vi "dl.vi"() -> ()   [LabVIEW 2025]
uses:
  <vilib>/Instr/_visa.llb/VISA Configure Serial Port (Instr).vi
panel:
  out "KONDENSATOR":dbl(slide) scale=2.8..3.3
  in  "?":bool
  in  "ILOŒÆ D¯ULI":dbl
  out "OSTATNI LOG":string
  out "LOGI":string[](array[string])
  in  "KONTRAST":dbl(knob) scale=0.0..1000.0
  in  "?":bool
  in  "?":bool
  in  "?":bool
  out "KONDENSATOR":dbl(graph)
  in  "stop":bool
  out "AKTUALNA WARTOŒÆ":dbl
  out "REZYSTOR":dbl(graph)
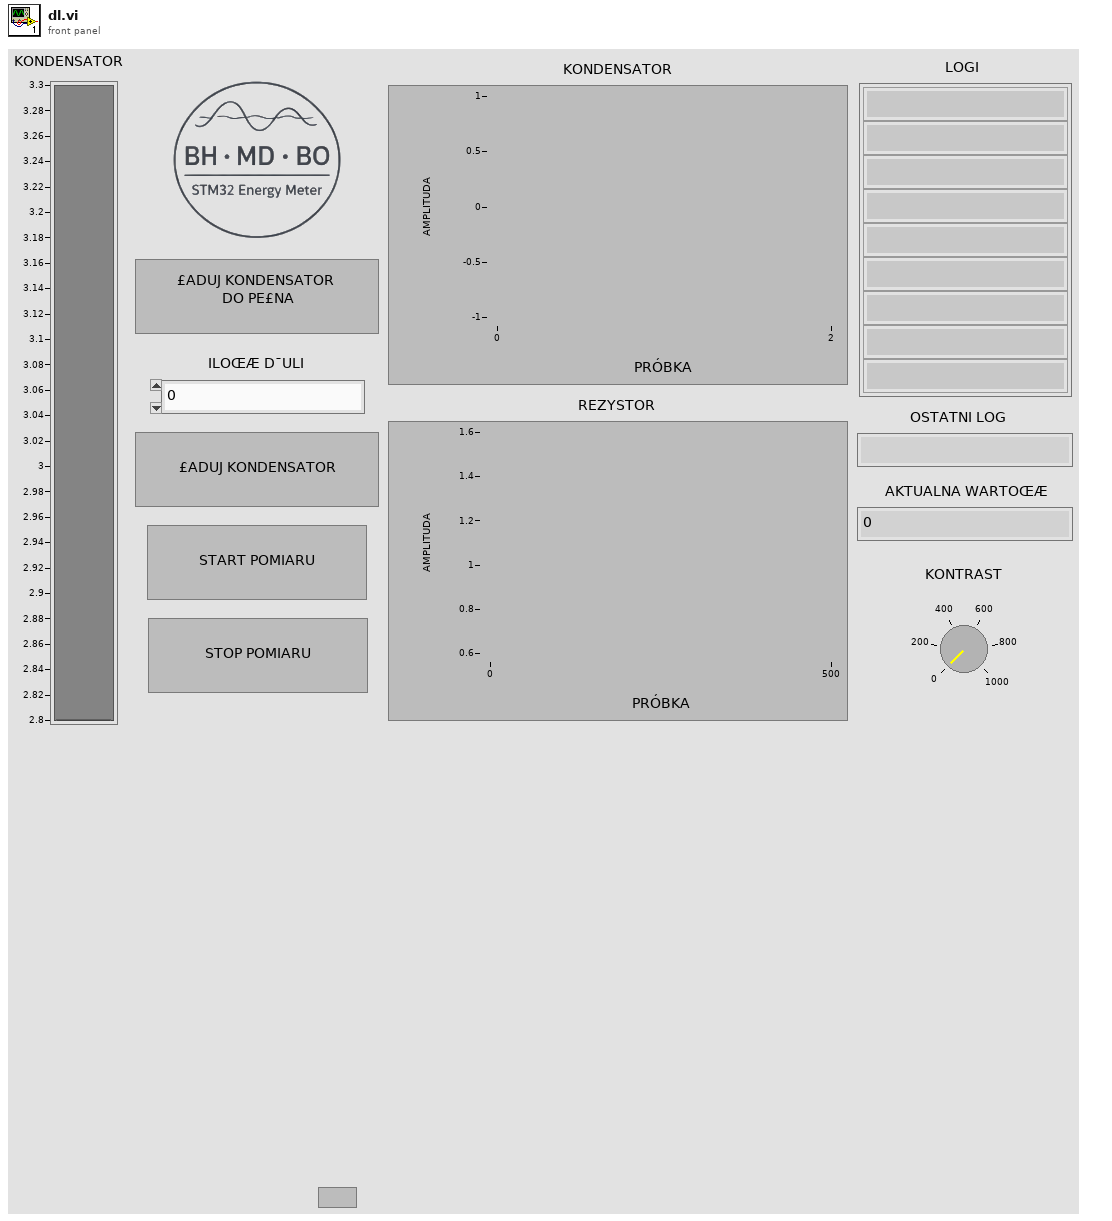
[diagram p1: front panel]
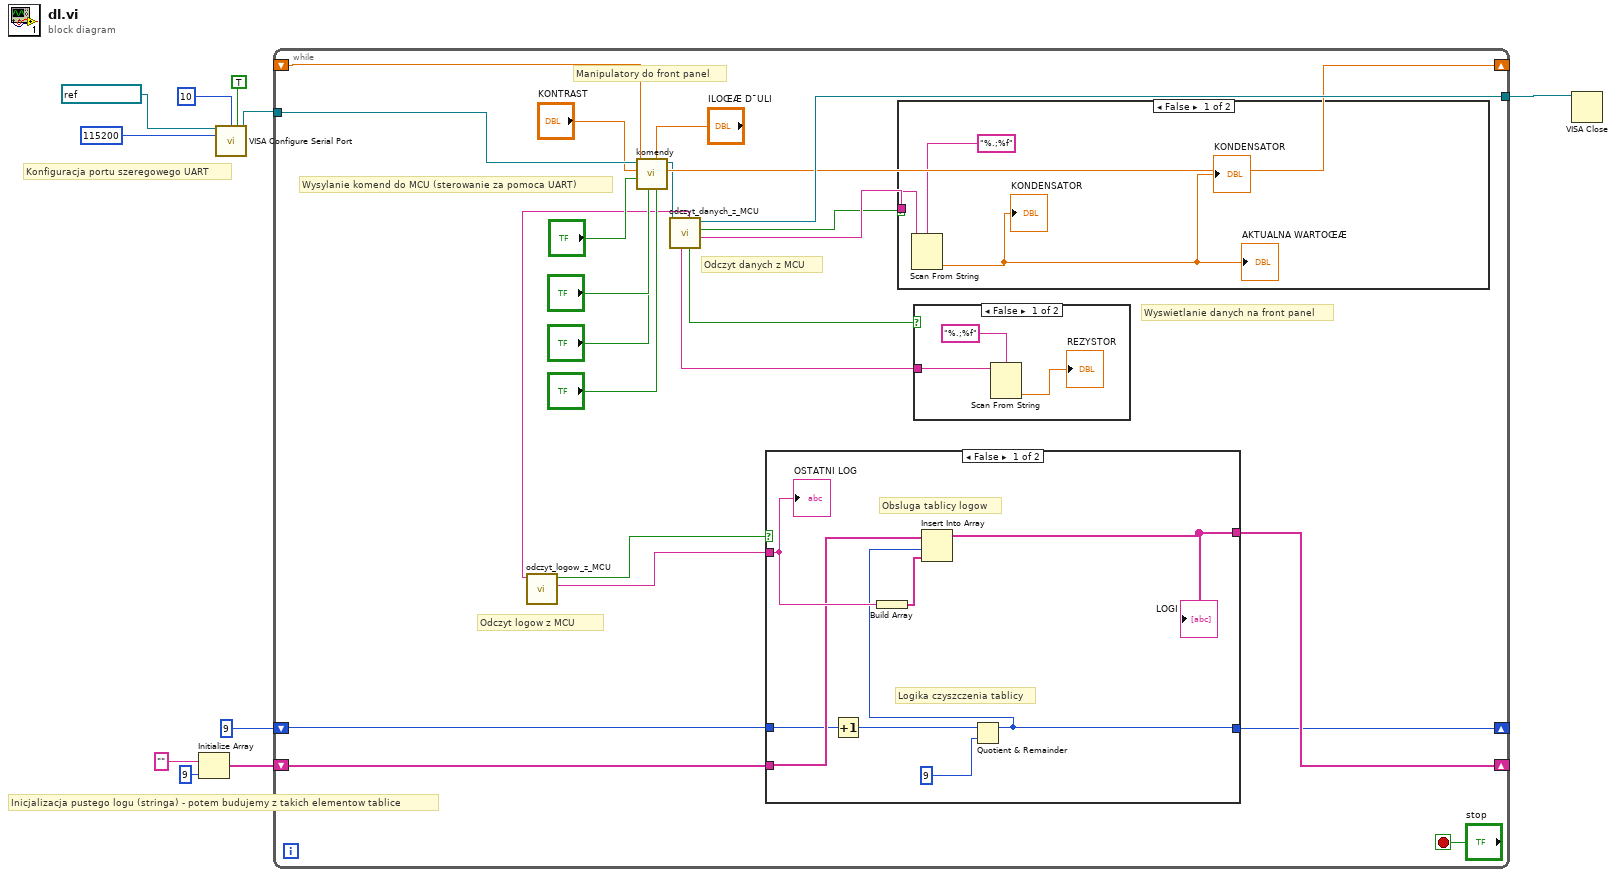
[diagram p0: block diagram]
diagram:
  # "Inicjalizacja pustego logu (stringa) - potem budujemy z takich elementow tablice"
  # "Konfiguracja portu szeregowego UART"
  n1 = Initialize Array("", 9 ("dimension size")) -> (w2:string[])
  n2 = call-poly "VISA Configure Serial Port"("VISA resource name"=refnum<visa-resource-name> "COM6", "termination char\n(0xA = '\\n' = LF)"=u8 10 ("termination char\n(0xA = '\\n' = LF)"), "Enable Termination\nChar (T)"=TRUE ("Enable Termination\nChar (T)"), "baud rate (9600)"=u32 115200) -> ("VISA resource name out"=w5:refnum<visa-resource-name>)  [unwired: 10 in, 1 out]
  n3 = while {
    tunnel: w5 -> [w19]
    tunnel: [w32] -> w6
    shift-right: [w23] -> _
    shift-left: _ -> [w24]
    shift-right: [w20] -> _
    shift-left: w2 -> [w17]
    shift-right: [w15] -> _
    shift-left: 9 ("y") -> [w16]
    stop <- "stop" stop-if-true
    # "Manipulatory do front panel"
    # "Wyswietlanie danych na front panel"
    # "Odczyt logow z MCU"
    # "Odczyt danych z MCU"
    # "Wysylanie komend do MCU (sterowanie za pomoca UART)"
    n4 = call "komendy.vi"(4:"?", "ILOŒÆ D¯ULI"="ILOŒÆ D¯ULI", 6:"?", 7:"?", "KONTRAST 3"=w24, 9:"?", "KONTRAST in"="KONTRAST", "VISA Refnum in"=w19) -> ("KONTRAST out"=w23:dbl, "VISA Refnum out"=w14:refnum<visa-resource-name>)  [unwired: 2 in]
    n5 = call "odczyt_danych_z_MCU.vi"("VISA Refnum in"=w14) -> ("read buffer 2"=w29:string, "Boolean"=w28:bool, "VISA Refnum out"=w32:refnum<visa-resource-name>, "Boolean 2"=w31:bool, "read buffer"=w18:string, "read buffer 3"=w30:string)  [unwired: 5 in]
    n6 = call "odczyt_logow_z_MCU.vi"("read buffer in"=w18) -> ("read buffer out"=w21:string, "Boolean"=w22:bool)  [unwired: 9 in]
    n7 = case shown="False" w22 {
      tunnel: w21 -> [w41 _]
      tunnel: [w34 w43] -> w20
      tunnel: w17 -> [w38 w43]
      tunnel: w16 -> [w36 w42]
      tunnel: [w35 w42] -> w15
      frame False {
        # "Logika czyszczenia tablicy"
        # "Obsluga tablicy logow"
        n8 = Increment(x=w36) -> (x+1=w37:i32)
        n9 = Build Array(w41) -> (w40:string[])
        n10 = Quotient & Remainder(x=w37, y=9) -> (x-y*floor(x/y)=w35:i32)  [unwired: 1 out]
        n11 = Insert Into Array(array=w38, index=w35, new element=w40) -> (w34:string[])
        "LOGI" <- w34
        "OSTATNI LOG" <- w41
      }
      frame True {
      }
    }
    n12 = case shown="False" w28 {
      tunnel: w29 -> [w45 _]
      frame False {
        n13 = Scan From String(format string="%.;%f", input string=w45) -> (output 1=→"AKTUALNA WARTOŒÆ" →"KONDENSATOR" →"KONDENSATOR":dbl)  [unwired: 3 in, 3 out]
      }
      frame True {
      }
    }
    n14 = case shown="False" w31 {
      tunnel: w30 -> [w47 _]
      frame False {
        n15 = Scan From String(format string="%.;%f", input string=w47) -> (output 1=→"REZYSTOR":dbl)  [unwired: 3 in, 3 out]
      }
      frame True {
      }
    }
  }
  n16 = VISA Close(VISA resource name=w6) -> ()  [unwired: 1 in, 1 out]
